vi "Frequency Linearization SubVI.vi"(0 "Triangolo dritto":bool=TRUE, 1 "Active PolyFit":bool, 2 "Sketri Input":dbl[](array[numeric])=[2047.0, 2034.0, 2021.0, 2008.0, 1995.0, 1982.0, 1969.0, 1956.0, 1943.0, 1930.0, 1917.0, 1904.0, 1891.0, 1879.0, 1866.0, 1853.0, 1840.0, 1827.0, 1815.0, 1802.0, 1789.0, 1777.0, 1764.0, 1751.0, 1739.0, 1726.0, 1714.0, 1701.0, 1689.0, 1676.0, 1664.0, 1651.0, 1639.0, 1626.0, 1614.0, 1602.0, 1589.0, 1577.0, 1565.0, 1552.0, 1540.0, 1528.0, 1516.0, 1503.0, 1491.0, 1479.0, 1467.0, 1455.0, 1443.0, 1431.0, 1419.0, 1407.0, 1395.0, 1383.0, 1371.0, 1359.0, 1347.0, 1335.0, 1323.0, 1311.0, 1299.0, 1287.0, 1276.0, 1264.0, 1252.0, 1240.0, 1229.0, 1217.0, 1205.0, 1194.0, 1182.0, 1170.0, 1159.0, 1147.0, 1136.0, 1124.0, 1113.0, 1101.0, 1090.0, 1078.0, 1067.0, 1055.0, 1044.0, 1033.0, 1021.0, 1010.0, 999.0, 987.0, 976.0, 965.0, 954.0, 942.0, 931.0, 920.0, 909.0, 898.0, 887.0, 876.0, 865.0, 854.0, 843.0, 832.0, 821.0, 810.0, 799.0, 788.0, 777.0, 766.0, 755.0, 744.0, 734.0, 723.0, 712.0, 701.0, 691.0, 685.0, 679.0, 674.0, 665.0, 658.0, 652.0, 647.0, 640.0, 634.0, 628.0, 618.0, 612.0, 605.0, 600.0, 594.0, 587.0, 582.0, 575.0, 570.0, 564.0, 559.0, 553.0, 548.0, 542.0, 537.0, 531.0, 525.0, 520.0, 514.0, 509.0, 503.0, 497.0, 492.0, 486.0, 480.0, 475.0, 469.0, 463.0, 458.0, 452.0, 446.0, 441.0, 435.0, 429.0, 423.0, 417.0, 411.0, 406.0, 400.0, 395.0, 389.0, 383.0, 377.0, 372.0, 366.0, 360.0, 355.0, 349.0, 344.0, 338.0, 333.0, 328.0, 322.0, 317.0, 311.0, 306.0, 300.0, 295.0, 289.0, 284.0, 278.0, 273.0, 268.0, 262.0, 257.0, 251.0, 246.0, 240.0, 235.0, 229.0, 224.0, 219.0, 213.0, 208.0, 202.0, 197.0, 191.0, 186.0, 181.0, 175.0, 170.0, 164.0, 159.0, 154.0, 148.0, 143.0, 137.0, 132.0, 127.0, 121.0, 116.0, 110.0, 105.0, 100.0, 94.0, 89.0, 84.0, 78.0, 73.0, 67.0, 62.0, 57.0, 51.0, 46.0, 41.0, 35.0, 30.0, 25.0, 19.0, 14.0, 8.0, 3.0, -3.0, -8.0, -13.0, -18.0, -24.0, -29.0, -35.0, -40.0, -45.0, -51.0, -56.0, -62.0, -67.0, -72.0, -78.0, -83.0, -88.0, -94.0, -99.0, -104.0, -110.0, -115.0, -120.0, -126.0, -131.0, -137.0, -142.0, -147.0, -153.0, -158.0, -163.0, -169.0, -174.0, -179.0, -185.0, -190.0, -195.0, -201.0, -206.0, -211.0, -217.0, -222.0, -227.0, -233.0, -238.0, -243.0, -249.0, -254.0, -259.0, -265.0, -270.0, -275.0, -281.0, -286.0, -291.0, -297.0, -302.0, -307.0, -313.0, -318.0, -323.0, -329.0, -334.0, -339.0, -345.0, -350.0, -355.0, -361.0, -366.0, -371.0, -377.0, -382.0, -387.0, -393.0, -398.0, -403.0, -408.0, -414.0, -419.0, -424.0, -430.0, -435.0, -440.0, -446.0, -451.0, -456.0, -462.0, -467.0, -472.0, -478.0, -483.0, -488.0, -494.0, -499.0, -504.0, -510.0, -515.0, -520.0, -526.0, -531.0, -536.0, -541.0, -547.0, -552.0, -557.0, -563.0, -568.0, -573.0, -579.0, -584.0, -589.0, -594.0, -600.0, -605.0, -610.0, -616.0, -621.0, -626.0, -631.0, -637.0, -642.0, -647.0, -652.0, -658.0, -663.0, -668.0, -673.0, -679.0, -684.0, -689.0, -695.0, -700.0, -705.0, -710.0, -716.0, -721.0, -726.0, -731.0, -737.0, -742.0, -747.0, -753.0, -758.0, -763.0, -768.0, -774.0, -779.0, -784.0, -789.0, -795.0, -800.0, -805.0, -811.0, -816.0, -821.0, -826.0, -832.0, -837.0, -842.0, -848.0, -853.0, -858.0, -864.0, -869.0, -874.0, -879.0, -885.0, -890.0, -895.0, -901.0, -906.0, -911.0, -916.0, -922.0, -927.0, -932.0, -938.0, -943.0, -948.0, -953.0, -959.0, -964.0, -969.0, -974.0, -980.0, -985.0, -990.0, -996.0, -1001.0, -1006.0, -1011.0, -1017.0, -1022.0, -1027.0, -1032.0, -1038.0, -1043.0, -1048.0, -1054.0, -1059.0, -1064.0, -1069.0, -1075.0, -1080.0, -1085.0, -1090.0, -1096.0, -1101.0, -1106.0, -1112.0, -1117.0, -1122.0, -1127.0, -1133.0, -1138.0, -1143.0, -1148.0, -1154.0, -1159.0, -1164.0, -1169.0, -1175.0, -1180.0, -1185.0, -1191.0, -1196.0, -1201.0, -1206.0, -1212.0, -1217.0, -1222.0, -1227.0, -1233.0, -1238.0, -1243.0, -1249.0, -1254.0, -1259.0, -1264.0, -1270.0, -1275.0, -1280.0, -1285.0, -1291.0, -1296.0, -1301.0, -1306.0, -1312.0, -1317.0, -1322.0, -1328.0, -1333.0, -1338.0, -1343.0, -1349.0, -1354.0, -1359.0, -1364.0, -1370.0, -1375.0, -1380.0, -1385.0, -1391.0, -1396.0, -1401.0, -1407.0, -1412.0, -1417.0, -1422.0, -1428.0, -1433.0, -1438.0, -1443.0, -1449.0, -1454.0, -1459.0, -1464.0, -1470.0, -1475.0, -1480.0, -1486.0, -1491.0, -1496.0, -1501.0, -1507.0, -1512.0, -1517.0, -1522.0, -1528.0, -1533.0, -1538.0, -1543.0, -1549.0, -1554.0, -1559.0, -1564.0, -1570.0, -1575.0, -1580.0, -1586.0, -1591.0, -1596.0, -1601.0, -1607.0, -1612.0, -1617.0, -1622.0, -1628.0, -1633.0, -1638.0, -1643.0, -1649.0, -1654.0, -1659.0, -1664.0, -1670.0, -1675.0, -1680.0, -1685.0, -1691.0, -1696.0, -1701.0, -1706.0, -1712.0, -1717.0, -1722.0, -1728.0, -1733.0, -1738.0, -1743.0, -1749.0, -1754.0, -1759.0, -1764.0, -1770.0, -1775.0, -1780.0, -1785.0, -1791.0, -1796.0, -1801.0, -1806.0, -1812.0, -1817.0, -1822.0, -1827.0, -1833.0, -1838.0, -1843.0, -1848.0, -1854.0, -1859.0, -1864.0, -1869.0, -1875.0, -1880.0, -1885.0, -1890.0, -1896.0, -1901.0, -1906.0, -1911.0, -1917.0, -1922.0, -1927.0, -1932.0, -1938.0, -1943.0, -1948.0, -1953.0, -1959.0, -1964.0, -1969.0, -1974.0, -1980.0, -1985.0, -1990.0, -1995.0, -2001.0, -2006.0, -2011.0, -2016.0, -2022.0, -2027.0, -2032.0, -2037.0, -2043.0, -2048.0, -2047.0, -2037.0, -2028.0, -2018.0, -2008.0, -1999.0, -1989.0, -1979.0, -1970.0, -1960.0, -1951.0, -1941.0, -1931.0, -1922.0, -1912.0, -1903.0, -1893.0, -1884.0, -1874.0, -1865.0, -1855.0, -1846.0, -1836.0, -1827.0, -1817.0, -1808.0, -1798.0, -1789.0, -1779.0, -1770.0, -1761.0, -1751.0, -1742.0, -1732.0, -1723.0, -1714.0, -1704.0, -1695.0, -1686.0, -1676.0, -1667.0, -1658.0, -1648.0, -1639.0, -1630.0, -1621.0, -1611.0, -1602.0, -1593.0, -1584.0, -1575.0, -1565.0, -1556.0, -1547.0, -1538.0, -1529.0, -1520.0, -1510.0, -1501.0, -1492.0, -1483.0, -1474.0, -1465.0, -1456.0, -1447.0, -1438.0, -1429.0, -1420.0, -1411.0, -1402.0, -1393.0, -1384.0, -1375.0, -1366.0, -1357.0, -1348.0, -1339.0, -1330.0, -1321.0, -1312.0, -1303.0, -1294.0, -1285.0, -1277.0, -1268.0, -1259.0, -1250.0, -1241.0, -1232.0, -1224.0, -1215.0, -1206.0, -1197.0, -1188.0, -1180.0, -1171.0, -1162.0, -1153.0, -1145.0, -1136.0, -1127.0, -1119.0, -1110.0, -1101.0, -1093.0, -1084.0, -1075.0, -1067.0, -1058.0, -1049.0, -1041.0, -1032.0, -1024.0, -1015.0, -1007.0, -998.0, -989.0, -981.0, -972.0, -964.0, -955.0, -909.0, -902.0, -894.0, -872.0, -865.0, -858.0, -850.0, -843.0, -836.0, -781.0, -774.0, -747.0, -740.0, -734.0, -727.0, -720.0, -714.0, -707.0, -700.0, -693.0, -687.0, -679.0, -672.0, -654.0, -647.0, -639.0, -632.0, -625.0, -619.0, -608.0, -601.0, -595.0, -588.0, -582.0, -575.0, -568.0, -562.0, -555.0, -549.0, -542.0, -535.0, -529.0, -522.0, -515.0, -509.0, -502.0, -496.0, -489.0, -482.0, -476.0, -469.0, -462.0, -456.0, -449.0, -441.0, -435.0, -427.0, -420.0, -413.0, -407.0, -401.0, -395.0, -387.0, -381.0, -373.0, -367.0, -361.0, -355.0, -349.0, -343.0, -337.0, -330.0, -324.0, -318.0, -312.0, -306.0, -300.0, -294.0, -288.0, -282.0, -276.0, -269.0, -263.0, -257.0, -251.0, -245.0, -239.0, -233.0, -227.0, -221.0, -215.0, -209.0, -203.0, -197.0, -191.0, -185.0, -179.0, -173.0, -167.0, -161.0, -155.0, -149.0, -143.0, -137.0, -131.0, -125.0, -119.0, -113.0, -107.0, -101.0, -95.0, -89.0, -83.0, -77.0, -71.0, -65.0, -59.0, -54.0, -48.0, -42.0, -36.0, -30.0, -23.0, -17.0, -11.0, -6.0, -0.0, 6.0, 13.0, 19.0, 25.0, 31.0, 37.0, 42.0, 48.0, 55.0, 61.0, 66.0, 72.0, 78.0, 84.0, 89.0, 95.0, 101.0, 106.0, 112.0, 118.0, 124.0, 129.0, 135.0, 141.0, 146.0, 152.0, 157.0, 163.0, 169.0, 174.0, 180.0, 186.0, 191.0, 197.0, 203.0, 208.0, 214.0, 219.0, 225.0, 231.0, 236.0, 242.0, 247.0, 253.0, 259.0, 264.0, 270.0, 275.0, 281.0, 287.0, 292.0, 298.0, 303.0, 309.0, 315.0, 320.0, 326.0, 331.0, 337.0, 343.0, 348.0, 354.0, 359.0, 365.0, 371.0, 376.0, 382.0, 387.0, 393.0, 399.0, 404.0, 410.0, 416.0, 421.0, 427.0, 433.0, 438.0, 444.0, 449.0, 455.0, 461.0, 466.0, 472.0, 477.0, 483.0, 488.0, 494.0, 500.0, 505.0, 511.0, 517.0, 522.0, 528.0, 533.0, 539.0, 544.0, 550.0, 555.0, 561.0, 566.0, 572.0, 577.0, 583.0, 588.0, 594.0, 599.0, 604.0, 610.0, 615.0, 621.0, 626.0, 632.0, 637.0, 643.0, 648.0, 654.0, 659.0, 665.0, 670.0, 675.0, 681.0, 686.0, 692.0, 697.0, 703.0, 708.0, 714.0, 719.0, 725.0, 730.0, 735.0, 741.0, 746.0, 752.0, 757.0, 763.0, 768.0, 774.0, 779.0, 785.0, 790.0, 795.0, 801.0, 806.0, 812.0, 817.0, 823.0, 828.0, 834.0, 839.0, 844.0, 850.0, 855.0, 861.0, 866.0, 872.0, 877.0, 882.0, 888.0, 893.0, 899.0, 904.0, 910.0, 915.0, 920.0, 926.0, 931.0, 937.0, 942.0, 947.0, 953.0, 958.0, 964.0, 969.0, 974.0, 980.0, 985.0, 991.0, 996.0, 1001.0, 1007.0, 1012.0, 1018.0, 1023.0, 1028.0, 1034.0, 1039.0, 1045.0, 1050.0, 1055.0, 1061.0, 1066.0, 1071.0, 1077.0, 1082.0, 1088.0, 1093.0, 1098.0, 1104.0, 1109.0, 1114.0, 1120.0, 1125.0, 1130.0, 1136.0, 1141.0, 1146.0, 1152.0, 1157.0, 1162.0, 1168.0, 1173.0, 1178.0, 1184.0, 1189.0, 1194.0, 1200.0, 1205.0, 1210.0, 1216.0, 1221.0, 1226.0, 1232.0, 1237.0, 1242.0, 1248.0, 1253.0, 1258.0, 1264.0, 1269.0, 1274.0, 1280.0, 1285.0, 1290.0, 1296.0, 1301.0, 1306.0, 1312.0, 1317.0, 1322.0, 1328.0, 1333.0, 1338.0, 1344.0, 1349.0, 1355.0, 1360.0, 1365.0, 1371.0, 1376.0, 1381.0, 1387.0, 1392.0, 1397.0, 1403.0, 1408.0, 1413.0, 1419.0, 1424.0, 1429.0, 1434.0, 1440.0, 1445.0, 1450.0, 1456.0, 1461.0, 1466.0, 1472.0, 1477.0, 1482.0, 1488.0, 1493.0, 1498.0, 1504.0, 1509.0, 1514.0, 1520.0, 1525.0, 1530.0, 1536.0, 1541.0, 1546.0, 1552.0, 1557.0, 1562.0, 1567.0, 1573.0, 1578.0, 1583.0, 1589.0, 1594.0, 1599.0, 1605.0, 1610.0, 1615.0, 1621.0, 1626.0, 1631.0, 1636.0, 1642.0, 1647.0, 1652.0, 1658.0, 1663.0, 1668.0, 1674.0, 1679.0, 1684.0, 1689.0, 1695.0, 1700.0, 1705.0, 1711.0, 1716.0, 1721.0, 1727.0, 1732.0, 1737.0, 1742.0, 1748.0, 1753.0, 1758.0, 1764.0, 1769.0, 1774.0, 1779.0, 1785.0, 1790.0, 1795.0, 1801.0, 1806.0, 1811.0, 1816.0, 1822.0, 1827.0, 1832.0, 1837.0, 1843.0, 1848.0, 1853.0, 1859.0, 1864.0, 1869.0, 1874.0, 1880.0, 1885.0, 1890.0, 1895.0, 1901.0, 1906.0, 1911.0, 1917.0, 1922.0, 1927.0, 1932.0, 1938.0, 1943.0, 1948.0, 1953.0, 1959.0, 1964.0, 1969.0, 1974.0, 1980.0, 1985.0, 1990.0, 1995.0, 2001.0, 2006.0, 2011.0, 2016.0, 2022.0, 2027.0, 2032.0, 2037.0, 2043.0, 2048.0], 3 "#Medie":i32=20, 5 "Scale factor":dbl(slide)=0.5 scale=0.01..1.0, 8 "Scaling factor":dbl=1.0, 10 "Sample /Modulation Frequency":enum32{"40MHz/32KHz", "30MHz/24Khz"}(radio)) -> (9 "Last Mean Freq Curve Rising":dbl[](graph), 11 "Last Mean Freq Curve Falling":dbl[](graph), 14 "Falling Std Dev %":dbl, 15 "Falling Max-Min error (% over Mean)":dbl, 16 "Rising Std Dev %":dbl, 17 "First Signal (Last)":dbl[](graph), 18 "Rising Max-Min error (% over Mean)":dbl, 19 "Second Signal (Last)":dbl[](graph))   [LabVIEW 2014]
uses:
  <vilib>/Platform/TimedLoop/XDataNode/timing_clust.ctl
  <vilib>/Platform/TimedLoop/XDataNode/nitl_modes.ctl
  <vilib>/Platform/TimedLoop/XDataNode/wakeup.ctl
  <vilib>/FPGAPlugInAG/sbRIO-9636/niLvFpga_Open_sbRIO-9636.vi
  <vilib>/rvi/interface/common/dynamic/niFpgaDynamicAddResources.vi
  <vilib>/Utility/error.llb/Error Cluster From Error Code.vi
  <vilib>/rvi/errors/niLvFpgaAdjustHostInterfaceError.vi
  <vilib>/rvi/interface/common/niFpgaWaitOnOcc.vi
  <vilib>/FPGAPlugInAG/Dynamic/niLvFpga_Run_Dynamic.vi
  <vilib>/FPGAPlugInAG/Dynamic/niLvFpga_Abort_Dynamic.vi
  <vilib>/FPGAPlugInAG/Dynamic/niLvFpga_Reset_Dynamic.vi
  <vilib>/FPGAPlugInAG/Dynamic/niLvFpga_Close_Dynamic.vi
  <vilib>/rvi/interface/nirviOpenFPGA/nirviOpenFPGA.xnode
  FPGA Bitfiles/LaserDistanceSen_FPGATarget_DoubleFFTMesuram_r82pz3ZO4sk.lvbitx
  FPGA Target/Test VIs/Double FFT Mesurament Test.vi
  FPGA Bitfiles/LaserDistanceSen_FPGATarget_DoubleFFTMesuram_atjrRfXVdPQ.lvbitx
  FPGA Target/Test VIs/Double FFT Mesurament Test SLOW.vi
  <vilib>/rvi/interface/nirviReadWriteControl/nirviReadWriteControl.xnode
  <vilib>/rvi/interface/nirviMethod/nirviMethod.xnode
  <vilib>/Platform/TimedLoop/XDataNode/XDataNode.xnode
  <vilib>/rvi/interface/nirviCloseFPGA/nirviCloseFPGA.xnode
  <vilib>/FPGAPlugInAG/Dynamic/niLvFpga_ConfigureFifo_Dynamic.vi
  <vilib>/rvi/errors/niLvFpgaMergeErrorWithErrorCode.vi
  <vilib>/FPGAPlugInAG/Dynamic/niLvFpga_StartFifo_Dynamic.vi
  <vilib>/rvi/interface/Simulation/niFpgaSimulationCallBeginRW.vi
  <vilib>/FPGAPlugInAG/Dynamic/niLvFpga_ReadFifo_Dynamic.vi
  <vilib>/Platform/TimedLoop/XDataNode/XDNodeRunTimeDep.lvlib
  NiFpgaLv.dll
panel:
  in  "Acrive  Smooth":bool
  out "Complete SkewTri":dbl[](graph)
  out "2) Tri edge RISING":dbl[](graph)
  out "1) Tri edge FALLING":dbl[](graph)
  out "1) Ext Mean Freq Curve":dbl[](graph)
  out "2) Ext Mean Freq Curve":dbl[](graph)
  out "2) Mean Freq Curve Rising":dbl[](graph)
  out "1) Mean Freq Curve Falling":dbl[](graph)
  out "2) Freq curve":dbl[](graph)
  out "1) Freq curve":dbl[](graph)
  in  "FFT Sliding Win Size":i32=128
  out "1) SmoothSubSig":dbl[](graph)
  out "2) SmoothSubSig":dbl[](graph)
  in  "Acrive Fit":bool=TRUE
  in  "Poly Order":i32=3
  in  "Side points":i32=13
  in  "Poly Grade":dbl=5.0
  out "2) Signal&Fit 2":dbl[][](graph)
  out "1) Signal&Fit":dbl[][](graph)
  out "Current Sig lin":i32
  in  "Acrive Linearization":bool=TRUE
  in  "?":bool
  out "maxbin_secondFFT":i32
  out "maxbin_firstFFT":i32
  out "f_rise":dbl
  out "f_fall":dbl
  out "f_mean":dbl
  out "Velocity (m/s)":dbl
  out "Distance (m)":dbl
  in  "Initial Latency points":u32(slide) scale=0.0..1249.0
  out "Second FFT (bin)":dbl[](graph)
  out "Second Signal (points) - Rising Triangular":dbl[](graph)
  out "First FFT (bin)":dbl[](graph)
  out "First Signal (points) - Falling Triangular":dbl[](graph)
  in  "Windowing":T1(ring)
  in  "first bin":i32=5
  in  "last bin":i32=255
  in  "lower limit 2":u32(slide)=738 scale=625.0..738.0
  in  "lower limit 1":u32(slide)=113 scale=0.0..113.0
  # "OFFLINE parameters"
  # "Triangolo storto\nda costante"
  # "Max Detection FFT bin range"
  # "ONLINE parameters"
  # "Se la sottrazione del fondo non è eseguita su FPGA.\n Attivarla per eseguirla lato RT"
  # "Smoothing (S-G Params)"
  # "Fitting"
  # "ONLY POWER OF 2"
  # "Min: 2 Max: 256 (2, 4, 8, 16, 32, 64, 128, 256)"
  # "LINEARIZATION FINAL RESULTS"
  # "%"
  # "%"
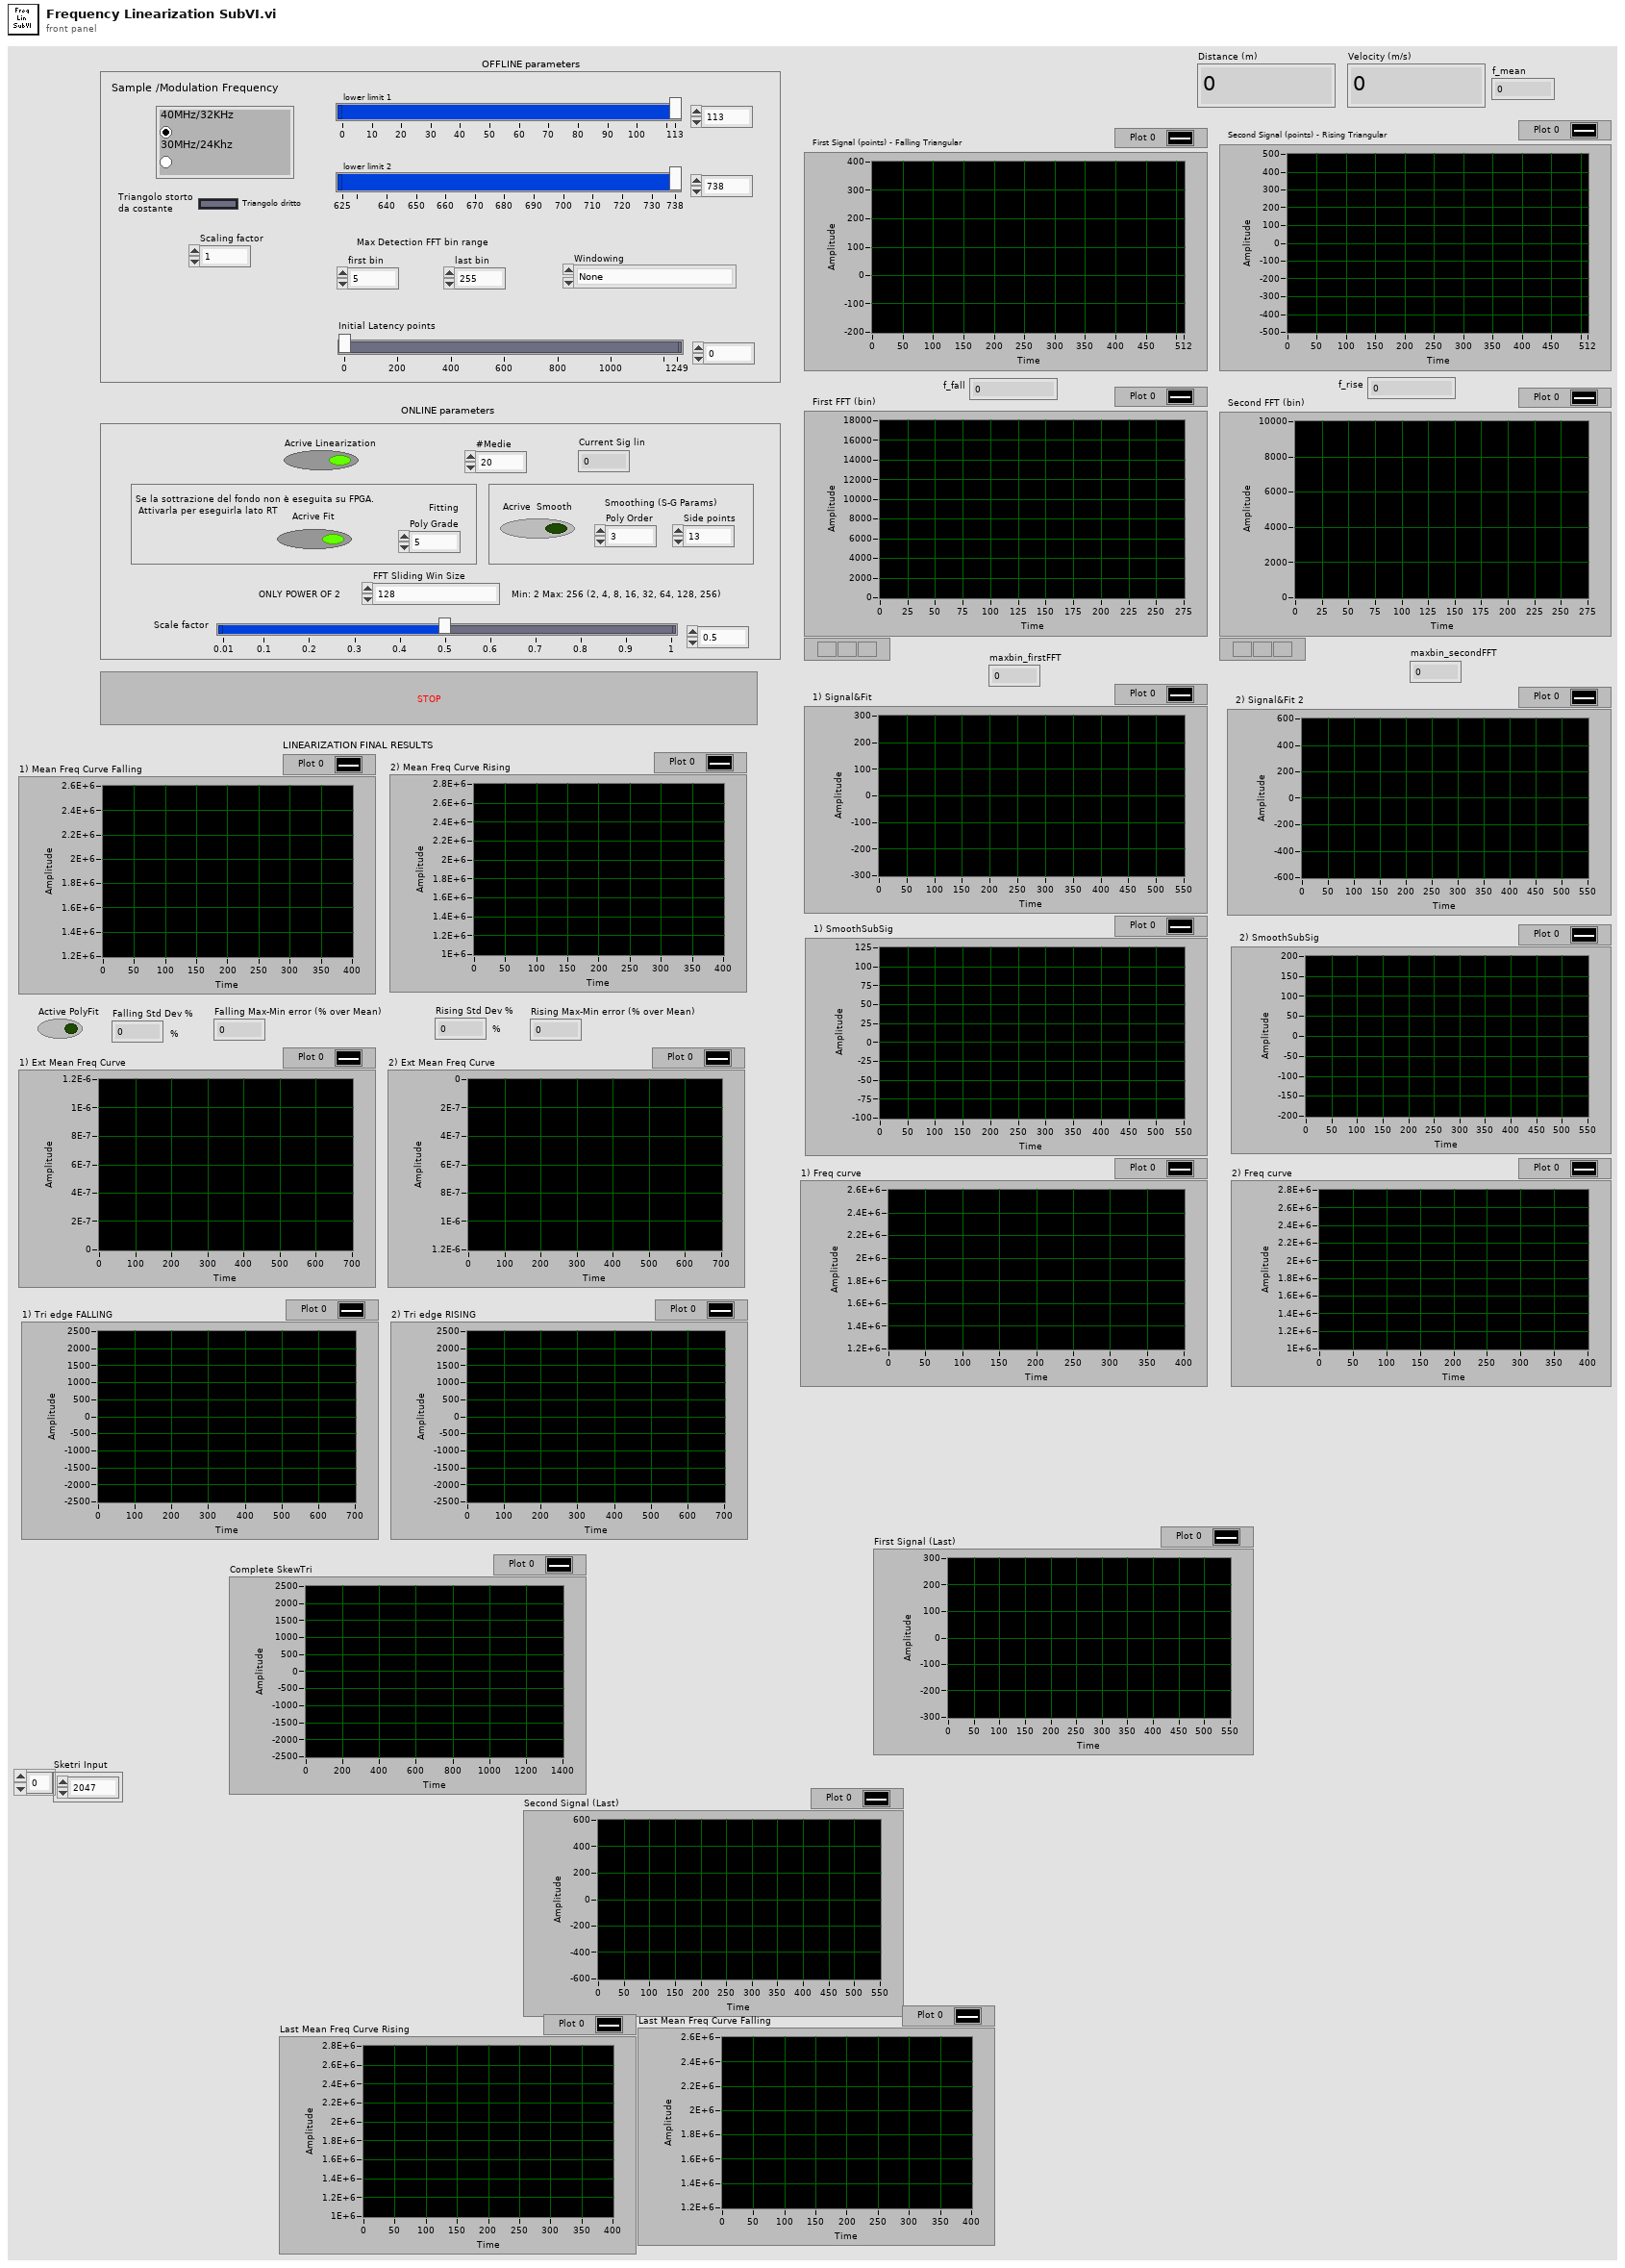
[diagram p1: front panel]
types:
  T1 = enum16{"None", "Hanning", "Hamming", "Blackman", "Blackman-Harris"}
  T2 = typedef "XDNodeRunTimeDep.lvlib/timing_clust.ctl" = cluster{"Expected End [f-1]":u64, "Actual End [f-1]":u64, "Finished Late? [f-1]":bool, "Expected End [i-1]":u64, "Actual End [i-1]":u64, "Finished Late? [i-1]":bool, "Expected Start [i]":u64, "Actual Start [i]":u64, "Expected Start [f]":u64, "Actual Start [f]":u64, "Source Name":string, "Structure Name":string, "Period":i64, "Deadline":i64, "Offset":i64, "Start":i64, "Priority":i32, "Timeout":i32, "Mode":T3, "Wakeup Reason":T4, "Error":errorcluster, "Source Type":string, "Secondary Source Type":string, "Global End Time":u64, "Global Start Time":u64, "Frame Duration":u64, "Iteration Duration":u64, "Assigned CPU":i32, "I/O Scan Engine Mode":u32}
  T3 = typedef "XDNodeRunTimeDep.lvlib/nitl_modes.ctl" = enum32{"No Change", "Process missed periods, maintain original phase", "Discard missed periods, maintain original phase", "Process missed periods, ignore original phase", "Discard missed periods, ignore original phase"}
  T4 = typedef "XDNodeRunTimeDep.lvlib/wakeup.ctl" = enum32{"Normal", "Aborted", "Asynchronous wakeup", "Timing source error", "Timed loop error", "Timeout"}
  T5 = typedef "NI_Matrix.lvlib/RealMatrix.ctl" = dbl[][]
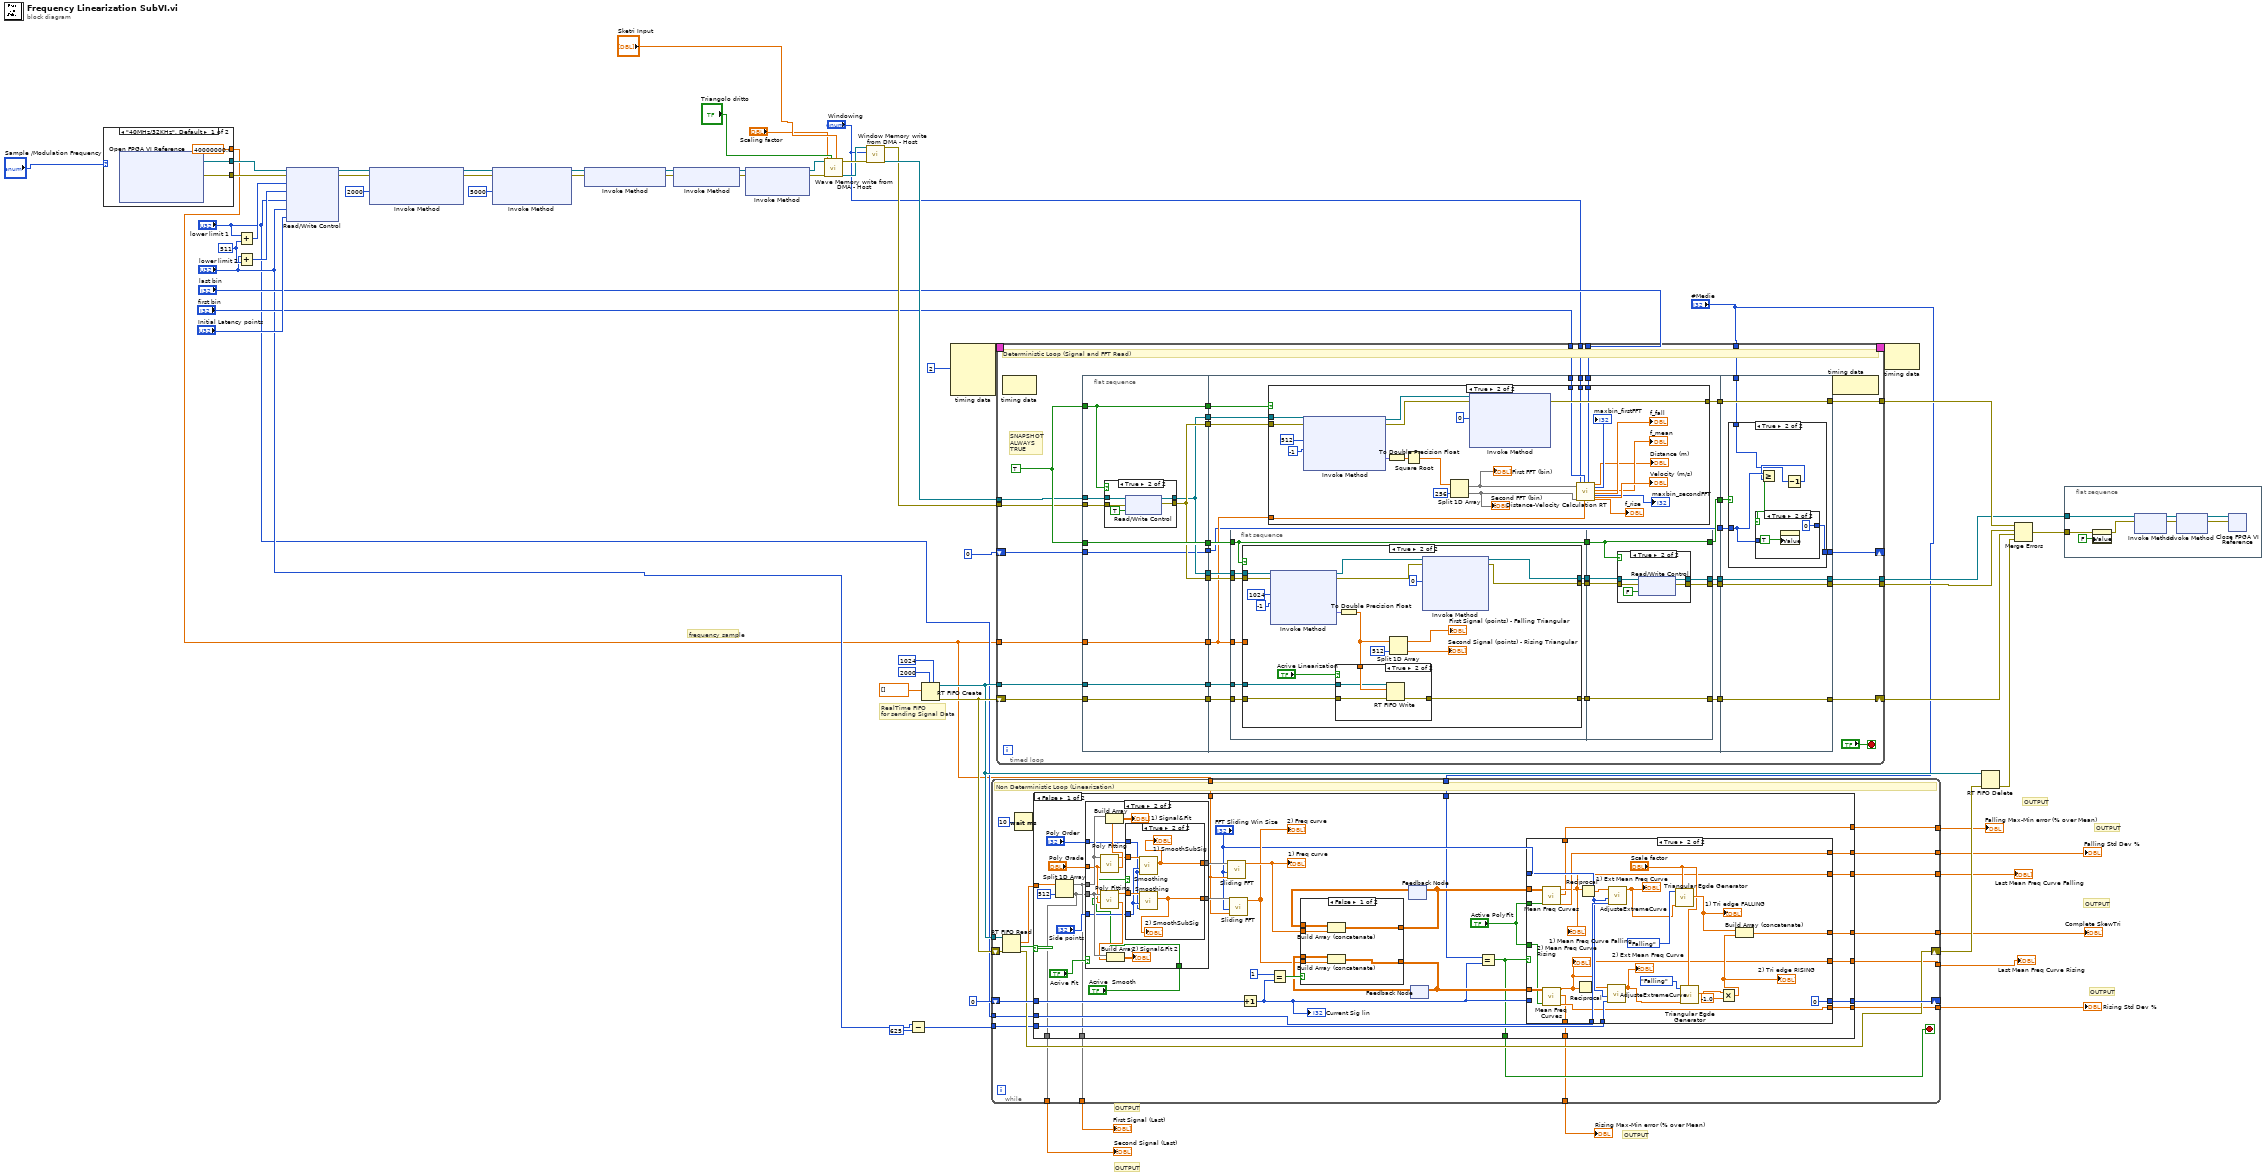
[diagram p0: block diagram]
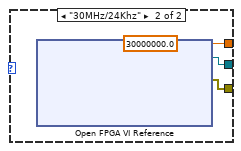
[diagram p2: hidden frame]
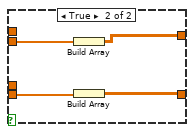
[diagram p6: hidden frame]
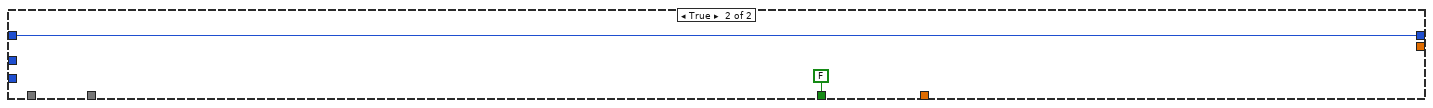
[diagram p7: hidden frame]
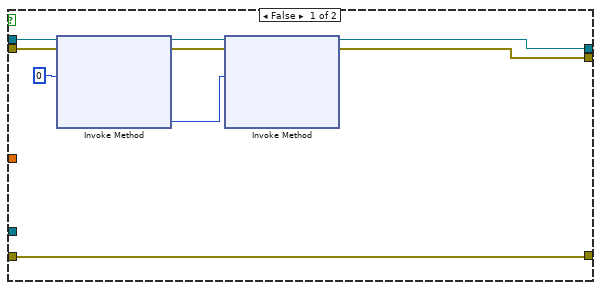
[diagram p9: hidden frame]
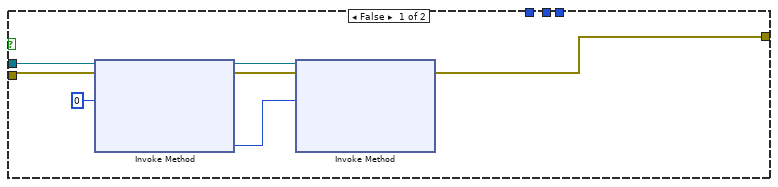
[diagram p12: hidden frame]
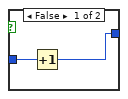
[diagram p14: hidden frame]
diagram:
  w61 = u32 511 ("y")
  # "OUTPUT"
  # "OUTPUT"
  # "frequency sample"
  # "OUTPUT"
  # "OUTPUT"
  # "OUTPUT"
  # "OUTPUT"
  # "OUTPUT"
  # "RealTime FIFO \nfor sending Signal Data"
  n1 = case shown="\"40MHz/32KHz\", Default" "Sample /Modulation Frequency" {
    tunnel: [w66 w67] -> w60
    tunnel: [w65 w68] -> w59
    tunnel: [40000000.0 30000000.0] -> w3
    frame "40MHz/32KHz", Default {
      n2 = xnode "Open FPGA VI Reference"() -> ("FPGA VI Reference Out"=w66:refnum<k20>, "error out"=w65:errorcluster)  [unwired: 2 in]
    }
    frame "30MHz/24Khz" {
      n3 = xnode "Open FPGA VI Reference"() -> ("FPGA VI Reference Out"=w67:refnum<k20>, "error out"=w68:errorcluster)  [unwired: 2 in]
    }
  }
  n4 = Add(x="lower limit 1", y=w61) -> (x+y=w63:u32)
  n5 = Add(x="lower limit 2", y=w61) -> (x+y=w62:u32)
  n6 = xnode "Read/Write Control"("FPGA VI Reference In"=w60, "error in"=w59, "upper limit 1"=w63, "upper limit 2"=w62, "lower limit 1"="lower limit 1", "lower limit 2"="lower limit 2", "Latency points"="Initial Latency points") -> ("FPGA VI Reference Out"=w56:refnum<k20>, "error out"=w55:errorcluster)
  n7 = xnode "Invoke Method"("FPGA VI Reference In"=w56, "error in"=w55, "Requested Depth"=u32 2000) -> ("FPGA VI Reference Out"=w34:refnum<k20>, "error out"=w35:errorcluster)  [unwired: 1 out]
  n8 = xnode "Invoke Method"("FPGA VI Reference In"=w34, "error in"=w35, "Requested Depth"=u32 5000) -> ("FPGA VI Reference Out"=w48:refnum<k20>, "error out"=w49:errorcluster)  [unwired: 1 out]
  n9 = xnode "Invoke Method"("FPGA VI Reference In"=w48, "error in"=w49) -> ("FPGA VI Reference Out"=w32:refnum<k20>, "error out"=w33:errorcluster)
  n10 = xnode "Invoke Method"("FPGA VI Reference In"=w32, "error in"=w33) -> ("FPGA VI Reference Out"=w46:refnum<k20>, "error out"=w47:errorcluster)
  n11 = xnode "Invoke Method"("FPGA VI Reference In"=w46, "error in"=w47) -> ("FPGA VI Reference Out"=w52:refnum<k20>, "error out"=w51:errorcluster)  [unwired: 1 in]
  n12 = call "Wave Memory write from DMA - Host.vi"("Custom Triangular Signal (fal-ris)"="Sketri Input", "Triangolo dritto?"="Triangolo dritto", "error in"=w51, "Scaling factor"="Scaling factor", "FPGA VI Reference In"=w52) -> ("FPGA VI Reference Out"=w37:refnum<k20>, "error out"=w50:errorcluster)  [unwired: 4 in, 1 out]
  n13 = call "Window Memory write from DMA - Host.vi"("error in"=w50, "Enum"="Windowing", "FPGA VI Reference In"=w37) -> ("FPGA VI Reference Out"=w58:refnum<k20>, "error out"=w57:errorcluster)  [unwired: 5 in, 2 out]
  n14 = Subtract(x="lower limit 2", y=u32 625) -> (x-y=w18:u32)
  n15 = RT FIFO Create(1:dbl[] [] ("double precision float"), 4:u32 2000 ("size (10)"), 6:u32 1024 ("elements in array (1)")) -> (8:w24:refnum<k33>, 11:w26:errorcluster)  [unwired: 5 in, 1 out]
  n16 = node-c288(i64 2 ("Period")) -> (w45:T2)  [unwired: 3 in]
  n17 = while {
    shift-right: [w84] -> w23
    shift-left: w26 -> [w86]
    tunnel: w24 -> [w90]
    shift-right: [w85] -> _
    shift-left: 0 -> [w89]
    tunnel: "lower limit 1" -> [w81]
    tunnel: w18 -> [w82]
    tunnel: w3 -> [w83]
    tunnel: [w80] -> w13
    tunnel: [w79] -> w12
    tunnel: [w78] -> w11
    tunnel: [w77] -> w10
    tunnel: [w76] -> w9
    tunnel: "#Medie" -> [w75]
    tunnel: [w73] -> w7
    tunnel: [w72] -> w6
    tunnel: [w71] -> w2
    tunnel: [w70] -> w1
    stop <- w74 stop-if-true
    # "Non Deterministic Loop (Linearization)"
    n18 = RT FIFO Read(0:w90, 3:w86) -> (9:w88:dbl[], 10:w87:bool, 11:w84:errorcluster)  [unwired: 2 in, 2 out]
    n19 = Wait (ms)(milliseconds to wait=u32 10 ("millisecond multiple")) -> ()  [unwired: 1 out]
    n20 = case shown="False" w87 {
      tunnel: w89 -> [w127 w190]
      tunnel: [w117 w190] -> w85
      tunnel: w88 -> [w125 _]
      tunnel: w83 -> [w110 _]
      tunnel: w82 -> [w107 _]
      tunnel: w81 -> [w106 _]
      tunnel: [w103 _] -> w80
      tunnel: [w102 _] -> w79
      tunnel: [w101 _] -> w78
      tunnel: [w100 _] -> w77
      tunnel: [w99 _] -> w76
      tunnel: w75 -> [w98 _]
      tunnel: [w97 FALSE] -> w74
      tunnel: [w96 _] -> w73
      tunnel: [w95 _] -> w72
      tunnel: [w93 _] -> w71
      tunnel: [w92 _] -> w70
      frame False {
        n21 = Split 1D Array(array=w125, index=512) -> (first subarray=w100:dbl[], second subarray=w99:dbl[])
        n22 = case shown="True" "Acrive Fit" {
          tunnel: w100 -> [w129 w143]
          tunnel: w99 -> [w128 w139]
          tunnel: "Poly Grade" -> [_ w135]
          tunnel: "Side points" -> [_ w134]
          tunnel: "Poly Order" -> [_ w133]
          tunnel: [w128 w132] -> w111
          tunnel: [w129 w130] -> w112
          tunnel: "Acrive  Smooth" -> [_ w131]
          frame False {
          }
          frame True {
            n23 = call "Poly Fitting.vi"("Poly Grade"=w135, "Signal"=w143) -> ("Poly Signal"=w142:dbl[], "SubtractedSignal"=w137:dbl[])  [unwired: 8 in]
            n24 = call "Poly Fitting.vi"("Poly Grade"=w135, "Signal"=w139) -> ("Poly Signal"=w138:dbl[], "SubtractedSignal"=w136:dbl[])  [unwired: 8 in]
            n25 = Build Array(w143, w142) -> (→"1) Signal&Fit":dbl[][])
            n26 = Build Array(w139, w138) -> (→"2) Signal&Fit 2":dbl[][])
            n27 = case shown="True" w131 {
              tunnel: w137 -> [w145 w151]
              tunnel: w136 -> [w144 w150]
              tunnel: w134 -> [_ w149]
              tunnel: w133 -> [_ w148]
              tunnel: [w144 w147] -> w132
              tunnel: [w145 w146] -> w130
              frame False {
              }
              frame True {
                n28 = call "Smoothing.vi"("polynomial order"=w148, "side points"=w149, "SubtractedSignal"=w151) -> ("SubSmoothSignal"=w146:dbl[])  [unwired: 8 in]
                "1) SmoothSubSig" <- w146
                n29 = call "Smoothing.vi"("polynomial order"=w148, "side points"=w149, "SubtractedSignal"=w150) -> ("SubSmoothSignal"=w147:dbl[])  [unwired: 8 in]
                "2) SmoothSubSig" <- w147
              }
            }
          }
        }
        n30 = call "Sliding FFT.vi"("Sample Freq"=w110, "FFT Win Size"="FFT Sliding Win Size", "SubSmoothSignal"=w112) -> ("Freq samples"=w109:dbl[])  [unwired: 7 in, 1 out]
        "1) Freq curve" <- w109
        n31 = call "Sliding FFT.vi"("Sample Freq"=w110, "FFT Win Size"="FFT Sliding Win Size", "SubSmoothSignal"=w111) -> ("Freq samples"=w108:dbl[])  [unwired: 7 in, 1 out]
        "2) Freq curve" <- w108
        n32 = Increment(x=w127) -> (x+1=w118:i32)
        "Current Sig lin" <- w118
        n33 = Equal?(x=1, y=w118) -> (x = y?=w123:bool)
        n34 = feedback #1() -> (w122:T5)  [unwired: 1 in]
        n35 = feedback #2() -> (w121:T5)  [unwired: 1 in]
        n36 = case shown="False" w123 {
          tunnel: w108 -> [w183 w186]
          tunnel: w109 -> [w184 w188]
          tunnel: [w182 w185] -> w119
          tunnel: [w181 w187] -> w120
          tunnel: w122 -> [w180 _]
          tunnel: w121 -> [w179 _]
          frame False {
            n37 = Build Array (concatenate)(w180, w184) -> (w181:T5)
            n38 = Build Array (concatenate)(w179, w183) -> (w182:T5)
          }
          frame True {
            n39 = Build Array(w188) -> (w187:T5)
            n40 = Build Array(w186) -> (w185:T5)
          }
        }
        n41 = feedback-in #1(w120) -> ()
        n42 = feedback-in #2(w119) -> ()
        n43 = Equal?(x=w98, y=w118) -> (x = y?=w97:bool)
        n44 = case shown="True" w97 {
          tunnel: w120 -> [_ w162]
          tunnel: w119 -> [_ w161]
          tunnel: w118 -> [w152 _]
          tunnel: [w152 0] -> w117
          tunnel: w107 -> [_ w174]
          tunnel: w106 -> [_ w173]
          tunnel: "FFT Sliding Win Size" -> [_ w172]
          tunnel: [_ w163] -> w103
          tunnel: [_ w158] -> w102
          tunnel: [_ w160] -> w101
          tunnel: [_ w157] -> w96
          tunnel: [_ w159] -> w95
          tunnel: "Active PolyFit" -> [_ w156]
          tunnel: "Active PolyFit" -> [_ w155]
          tunnel: [_ w154] -> w93
          tunnel: [_ w153] -> w92
          frame False {
          }
          frame True {
            n45 = call "Mean Freq Curves.vi"("Set of Freq samples"=w161, "Active Fit"=w155) -> ("Mean Freq Curve"=w159:dbl[], "Max-Min error (% over Mean)"=w154:dbl, "StdDev%"=w160:dbl)  [unwired: 12 in, 3 out]
            "2) Mean Freq Curve Rising" <- w159
            n46 = call "Mean Freq Curves.vi"("Set of Freq samples"=w162, "Active Fit"=w156) -> ("Mean Freq Curve"=w157:dbl[], "Max-Min error (% over Mean)"=w153:dbl, "StdDev%"=w158:dbl)  [unwired: 12 in, 3 out]
            "1) Mean Freq Curve Falling" <- w157
            n47 = Reciprocal(x=w159) -> (1/x=w169:dbl[])
            n48 = Reciprocal(x=w157) -> (1/x=w168:dbl[])
            n49 = call "AdjusteExtremeCurve.vi"("Init Bins Discarded"=w174, "FFT Size Window"=w172, "Freq sample"=w169) -> ("Extended Freq Sample"=w170:dbl[])  [unwired: 8 in]
            "2) Ext Mean Freq Curve" <- w170
            n50 = call "AdjusteExtremeCurve.vi"("Init Bins Discarded"=w173, "FFT Size Window"=w172, "Freq sample"=w168) -> ("Extended Freq Sample"=w171:dbl[])  [unwired: 8 in]
            "1) Ext Mean Freq Curve" <- w171
            n51 = call "Triangular Egde Generator.vi"("fattore"="Scale factor", "Sample values"=w171, "Triangular edge"=enum16{"Rising", "Falling"}."Falling") -> ("Skew Triangular"=w175:dbl[])  [unwired: 8 in]
            "1) Tri edge FALLING" <- w175
            n52 = call "Triangular Egde Generator.vi"("fattore"="Scale factor", "Sample values"=w170, "Triangular edge"=enum16{"Rising", "Falling"}."Falling") -> ("Skew Triangular"=w166:dbl[])  [unwired: 8 in]
            n53 = Multiply(x=w166, y=-1.0) -> (x*y=w165:dbl[])
            "2) Tri edge RISING" <- w165
            n54 = Build Array (concatenate)(w175, w165) -> (w163:dbl[])
          }
        }
      }
      frame True {
      }
    }
  }
  "Complete SkewTri" <- w13
  "Falling Std Dev %" <- w12
  "Rising Std Dev %" <- w11
  "First Signal (Last)" <- w10
  "Second Signal (Last)" <- w9
  "Last Mean Freq Curve Falling" <- w7
  "Last Mean Freq Curve Rising" <- w6
  "Rising Max-Min error (% over Mean)" <- w2
  "Falling Max-Min error (% over Mean)" <- w1
  n55 = timed-loop {
    tunnel: w58 -> [w218]
    tunnel: w57 -> [w219]
    tunnel: [w221] -> w42
    tunnel: w3 -> [w223]
    tunnel: [w222] -> w41
    timing: w45 -> [_]
    timing-out: [_] -> w44
    tunnel: "first bin" -> [w207]
    tunnel: "last bin" -> [w206]
    tunnel: [w204] -> w36
    tunnel: "Windowing" -> [w202]
    shift-right: [w196] -> w27
    shift-left: w26 -> [w198]
    tunnel: w24 -> [w200]
    shift-right: [w192] -> _
    shift-left: 0 -> [w194]
    tunnel: "#Medie" -> [w191]
    stop <- "?" stop-if-true
    w220 = TRUE ("Snapshot")
    # "SNAPSHOT\nALWAYS\nTRUE"
    # "Deterministic Loop (Signal and FFT Read)"
    n56 = node-c288() -> ()  [unwired: 1 in, 1 out]
    n57 = flat-sequence {
      tunnel: w218 -> [w231]
      tunnel: w219 -> [w232]
      tunnel: w220 -> [w229]
      tunnel: w220 -> [w234]
      tunnel: w223 -> [w235]
      tunnel: [w233] -> w217
      tunnel: [w235] -> w216
      tunnel: [w234] -> w215
      tunnel: [w229] -> w214
      tunnel: [w233] -> w213
      tunnel: [w230] -> w212
      tunnel: [w230] -> w211
      tunnel: [w228] -> w201
      tunnel: w200 -> [w228]
      tunnel: [w227] -> w199
      tunnel: w198 -> [w227]
      tunnel: [w226] -> w195
      tunnel: w194 -> [w226]
      tunnel: w217 -> [w260]
      tunnel: w216 -> [w248]
      tunnel: w215 -> [w254]
      tunnel: w214 -> [w257]
      tunnel: w213 -> [w256]
      tunnel: w212 -> [w255]
      tunnel: w211 -> [w261]
      tunnel: [w259] -> w210
      tunnel: [w258] -> w209
      tunnel: [w253] -> w208
      tunnel: w207 -> [w252]
      tunnel: w206 -> [w251]
      tunnel: [w250] -> w203
      tunnel: w202 -> [w249]
      tunnel: w201 -> [w247]
      tunnel: w199 -> [w246]
      tunnel: [w244] -> w197
      tunnel: w195 -> [w243]
      tunnel: [w243] -> w193
      tunnel: [w357] -> w221
      tunnel: [w358] -> w222
      tunnel: w210 -> [w358]
      tunnel: w209 -> [w357]
      tunnel: w208 -> [w356]
      tunnel: [w355] -> w204
      tunnel: w203 -> [w355]
      tunnel: [w354] -> w196
      tunnel: w197 -> [w354]
      tunnel: w193 -> [w353]
      tunnel: [w352] -> w192
      tunnel: w191 -> [w351]
      frame #0 {
        n58 = case shown="True" w229 {
          tunnel: [w236 w241] -> w233
          tunnel: w232 -> [w236 w240]
          tunnel: w231 -> [w237 w239]
          tunnel: [w237 w238] -> w230
          frame False {
          }
          frame True {
            n59 = xnode "Read/Write Control"("FPGA VI Reference In"=w239, "error in"=w240, "snapshot"=TRUE) -> ("FPGA VI Reference Out"=w238:refnum<k20>, "error out"=w241:errorcluster)
          }
        }
      }
      frame #1 {
        n60 = flat-sequence {
          tunnel: w261 -> [w273]
          tunnel: w260 -> [w272]
          tunnel: w248 -> [w271]
          tunnel: w254 -> [w268]
          tunnel: [w270] -> w264
          tunnel: [w269] -> w263
          tunnel: [w268] -> w262
          tunnel: w247 -> [w267]
          tunnel: w246 -> [w266]
          tunnel: [w265] -> w245
          tunnel: [w309] -> w258
          tunnel: w264 -> [w311]
          tunnel: w263 -> [w310]
          tunnel: w262 -> [w308]
          tunnel: [w308] -> w253
          tunnel: [w307] -> w250
          tunnel: [w306] -> w244
          tunnel: w245 -> [w306]
          frame #0 {
            n61 = case shown="True" w268 {
              tunnel: w273 -> [w281 w300]
              tunnel: w272 -> [w279 w299]
              tunnel: [w278 w292] -> w269
              tunnel: w271 -> [_ _]
              tunnel: [w275 w291] -> w270
              tunnel: w267 -> [_ w286]
              tunnel: w266 -> [w274 w285]
              tunnel: [w274 w284] -> w265
              frame False {
                n62 = xnode "Invoke Method"("FPGA VI Reference In"=w281, "error in"=w279, "Number of Elements"=u32 0) -> ("FPGA VI Reference Out"=w277:refnum<k20>, "error out"=w276:errorcluster, "Elements Remaining"=w280:u32)  [unwired: 1 in, 1 out]
                n63 = xnode "Invoke Method"("FPGA VI Reference In"=w277, "error in"=w276, "Number of Elements"=w280) -> ("FPGA VI Reference Out"=w275:refnum<k20>, "error out"=w278:errorcluster)  [unwired: 1 in, 2 out]
              }
              frame True {
                n64 = xnode "Invoke Method"("FPGA VI Reference In"=w300, "error in"=w299, "Number of Elements"=u32 1024, "Timeout (ms)"=-1) -> ("FPGA VI Reference Out"=w294:refnum<k20>, "error out"=w293:errorcluster, "Data"=w296:fxp<+/-,12,12>[])  [unwired: 1 out]
                n65 = To Double Precision Float(number=w296) -> (double precision float=w287:dbl[])
                n66 = case shown="True" "Acrive Linearization" {
                  tunnel: w287 -> [_ w305]
                  tunnel: w286 -> [_ w304]
                  tunnel: w285 -> [w301 w303]
                  tunnel: [w301 w302] -> w284
                  frame False {
                  }
                  frame True {
                    n67 = RT FIFO Write(0:w304, 1:w305, 3:w303) -> (11:w302:errorcluster)  [unwired: 2 in, 3 out]
                  }
                }
                n68 = Split 1D Array(array=w287, index=512) -> (first subarray=→"First Signal (points) - Falling Triangular":dbl[], second subarray=→"Second Signal (points) - Rising Triangular":dbl[])
                n69 = xnode "Invoke Method"("FPGA VI Reference In"=w294, "error in"=w293, "Number of Elements"=u32 0) -> ("FPGA VI Reference Out"=w291:refnum<k20>, "error out"=w292:errorcluster)  [unwired: 1 in, 2 out]
              }
            }
          }
          frame #1 {
            n70 = case shown="True" w308 {
              tunnel: [w313 w316] -> w309
              tunnel: w311 -> [w312 w317]
              tunnel: w310 -> [w313 w315]
              tunnel: [w312 w314] -> w307
              frame False {
              }
              frame True {
                n71 = xnode "Read/Write Control"("FPGA VI Reference In"=w317, "error in"=w315, "snapshot"=FALSE) -> ("FPGA VI Reference Out"=w314:refnum<k20>, "error out"=w316:errorcluster)
              }
            }
          }
        }
        n72 = case shown="True" w257 {
          tunnel: w255 -> [w324 w345]
          tunnel: w256 -> [w321 w346]
          tunnel: [w320 w344] -> w259
          tunnel: w252 -> [_ w331]
          tunnel: w251 -> [_ w332]
          tunnel: w249 -> [_ w328]
          tunnel: w248 -> [_ w326]
          frame False {
            n73 = xnode "Invoke Method"("FPGA VI Reference In"=w324, "error in"=w321, "Number of Elements"=u32 0) -> ("FPGA VI Reference Out"=w322:refnum<k20>, "error out"=w319:errorcluster, "Elements Remaining"=w323:u32)  [unwired: 1 in, 1 out]
            n74 = xnode "Invoke Method"("FPGA VI Reference In"=w322, "error in"=w319, "Number of Elements"=w323) -> ("error out"=w320:errorcluster)  [unwired: 1 in, 3 out]
          }
          frame True {
            n75 = xnode "Invoke Method"("FPGA VI Reference In"=w345, "error in"=w346, "Number of Elements"=u32 512, "Timeout (ms)"=-1) -> ("FPGA VI Reference Out"=w342:refnum<k20>, "error out"=w343:errorcluster, "Data"=w348:fxp<+,44,44>[])  [unwired: 1 out]
            n76 = To Double Precision Float(number=w348) -> (double precision float=w347:dbl[])
            n77 = Square Root(x=w347) -> (sqrt(x)=w340:dbl[])
            n78 = Split 1D Array(array=w340, index=256) -> (first subarray=w338:dbl[], second subarray=w337:dbl[])
            "First FFT (bin)" <- w338
            "Second FFT (bin)" <- w337
            n79 = xnode "Invoke Method"("FPGA VI Reference In"=w342, "error in"=w343, "Number of Elements"=u32 0) -> ("error out"=w344:errorcluster)  [unwired: 1 in, 3 out]
            n80 = call "Distance-Velocity Calculation RT.vi"("First FFT"=w338, "Second FFT"=w337, "Windowing"=w328, "first FFT bin"=w331, "Sample Rate (S/s)"=w326, "last FFT bin"=w332) -> ("F_rise"=→"f_rise":dbl, "maxbin_firstFFT"=→"maxbin_firstFFT":i32, "maxbin_secondFFT"=→"maxbin_secondFFT":i32, "Distance (m)"=→"Distance (m)":dbl, "f_mean"=→"f_mean":dbl, "F_fall"=→"f_fall":dbl, "Velocity (m/s)"=→"Velocity (m/s)":dbl)  [unwired: 7 in]
          }
        }
      }
      frame #2 {
        n81 = case shown="True" w356 {
          tunnel: w353 -> [w359 w363]
          tunnel: [w359 w364] -> w352
          tunnel: w351 -> [_ w360]
          frame False {
          }
          frame True {
            n82 = Decrement(x=w360) -> (x-1=w361:i32)
            n83 = Greater Or Equal?(x=w363, y=w361) -> (x >= y?=w362:bool)
            n84 = case shown="True" w362 {
              tunnel: w363 -> [w365 _]
              tunnel: [w366 0] -> w364
              frame False {
                n85 = Increment(x=w365) -> (x+1=w366:i32)
              }
              frame True {
                n86 = property class="Bool (strict)"("Value"=TRUE ("Snapshot")) -> ()  [unwired: 2 in, 2 out]
              }
            }
          }
        }
      }
    }
    n87 = node-c288() -> ()  [unwired: 1 in, 1 out]
  }
  n88 = node-c288(w44) -> ()  [unwired: 1 out]
  n89 = RT FIFO Delete(0:w24, 3:w23) -> (11:w22:errorcluster)  [unwired: 1 in]
  n90 = Merge Errors(w41, w42, w27, w22) -> (w25:errorcluster)
  n91 = flat-sequence {
    tunnel: w25 -> [w372]
    tunnel: w36 -> [w369]
    frame #0 {
      n92 = property class="Bool (strict)"(error in=w372, "Value"=FALSE ("stop")) -> (error out=w371:errorcluster)  [unwired: 1 in, 1 out]
      n93 = xnode "Invoke Method"("FPGA VI Reference In"=w369, "error in"=w371) -> ("FPGA VI Reference Out"=w374:refnum<k20>, "error out"=w373:errorcluster)
      n94 = xnode "Invoke Method"("FPGA VI Reference In"=w374, "error in"=w373) -> ("FPGA VI Reference Out"=w375:refnum<k20>, "error out"=w376:errorcluster)
      n95 = xnode "Close FPGA VI Reference"("FPGA VI Reference In"=w375, "error in"=w376) -> ()  [unwired: 1 out]
    }
  }
